vi "Update LCD.vi"(8 "error in":errorcluster, 11 "Front Panel Private Data in":T1) -> (0 "error out":errorcluster, 3 "LCD":string)   [LabVIEW 2026]
uses:
  controls/Front Panel Private Data.ctl
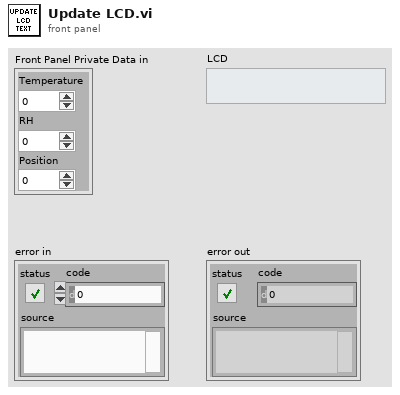
[diagram p1: front panel]
types:
  T1 = typedef "Front Panel Private Data.ctl" = cluster{"Temperature":dbl, "RH":dbl, "Position":dbl}
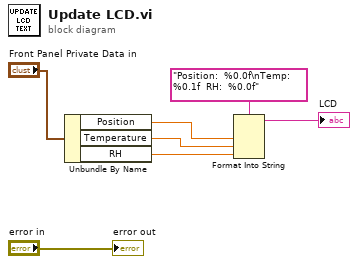
[diagram p0: block diagram]
diagram:
  n1 = Unbundle By Name("Front Panel Private Data in") -> ("Position"=w4:dbl, "Temperature"=w5:dbl, "RH"=w6:dbl)
  n2 = Format Into String(format string="Position:  %0.0f\nTemp:  %0.1f  RH:  %0.0f", w4, w5, w6) -> (resulting string=→"LCD":string)  [unwired: 2 in, 1 out]
  "error out" <- "error in"
